vi "Get BLISS_Create Full Path.vi"(8 "error in":errorcluster, 11 "Path to Create":path=path "C:/Users/Public/Documents/National Instruments/BLISS Image Sampler") -> (0 "error out":errorcluster, 2 "Folders Created":string[](array[string]), 3 "Path Out":path)   [LabVIEW 2020]
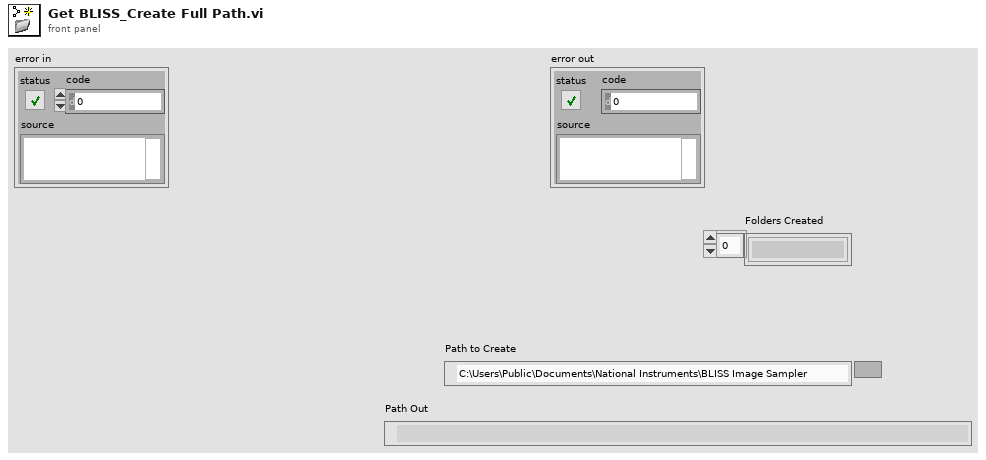
[diagram p1: front panel]
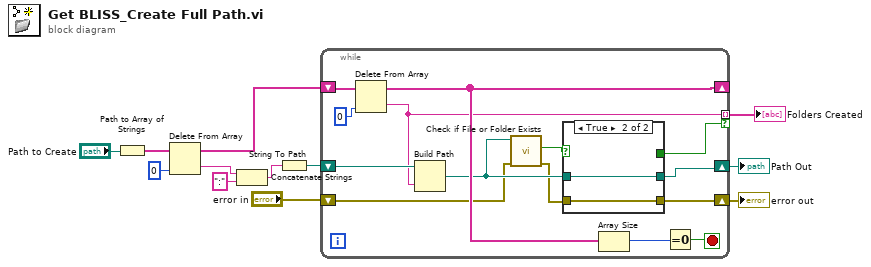
[diagram p0: block diagram]
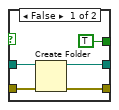
[diagram p2: hidden frame]
diagram:
  n1 = Path to Array of Strings(0:"Path to Create") -> (2:w11:string[])  [unwired: 1 out]
  n2 = Delete From Array(array=w11, index=0) -> (deleted portion=w7:string, array with subset deleted=w10:string[])  [unwired: 1 in]
  n3 = Concatenate Strings(w7, ":" ("string")) -> (w5:string)
  n4 = String To Path(string=w5) -> (path=w9:path)
  n5 = while {
    shift-right: [w18] -> w1
    shift-left: w9 -> [w26]
    shift-right: [w22] -> _
    shift-left: w10 -> [w25]
    tunnel: [w17] -> w4 mode=indexing if=w16
    shift-right: [w14] -> w2
    shift-left: "error in" -> [w13]
    stop <- w23 stop-if-true
    n6 = Delete From Array(array=w25, index=0) -> (deleted portion=w17:string, array with subset deleted=w22:string[])  [unwired: 1 in]
    n7 = Build Path(base path=w26, name or relative path=w17) -> (appended path=w20:path)
    n8 = call <vilib>:"Check if File or Folder Exists.vi"("error in (no error)"=w13, "path"=w20) -> ("error out"=w15:errorcluster, "file or folder exists?"=w19:bool)  [unwired: 7 in, 1 out]
    n9 = case shown="True" w19 {
      tunnel: w20 -> [w31 w33]
      tunnel: [w30 w33] -> w18
      tunnel: [TRUE _] -> w16
      tunnel: w15 -> [w28 w32]
      tunnel: [w27 w32] -> w14
      frame False {
        n10 = Create Folder(path (use dialog)=w31, error in=w28) -> (created path=w30:path, error out=w27:errorcluster)  [unwired: 1 in, 1 out]
      }
      frame True {
      }
    }
    n11 = Array Size(array=w22) -> (size(s)=w24:i32)
    n12 = Equal To 0?(x=w24) -> (x = 0?=w23:bool)
  }
  "Folders Created" <- w4
  "error out" <- w2
  "Path Out" <- w1
